vi "initialise.vi"(8 "error in (no error)":errorcluster, 11 "GenericPlugin in":refnum<class "TrajectoryMG100122GenericFPGA.lvclass">) -> (0 "error out":errorcluster, 3 "GenericPlugin out":refnum<class "TrajectoryMG100122GenericFPGA.lvclass">)   [LabVIEW 2010, in "TrajectoryMG100122GenericFPGA.lvclass"]
doc: "The dynamic dispatch-version of this VI initalises the plug-in object by allocating and initalising any dynamic resources need."
uses:
  TrajectoryMG100122GenericFPGA.lvclass
  GenericTrajectory/GenericTrajectory/GenericTrajectory.lvclass
  FPGAWrapper/GenericFPGAWrapper/GenericFPGAWrapper/GenericFPGAWrapper.lvclass
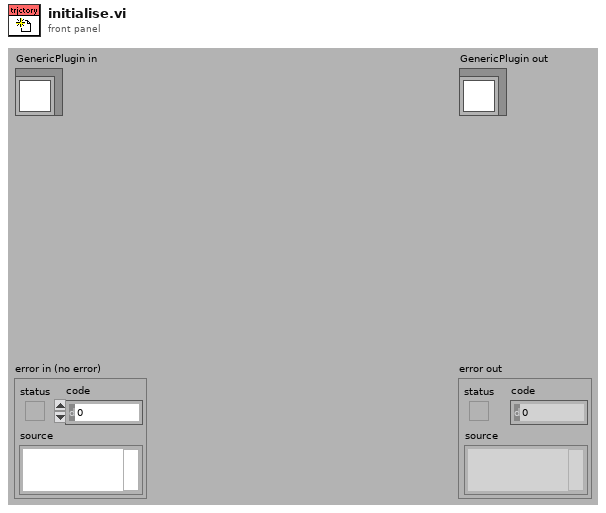
[diagram p1: front panel]
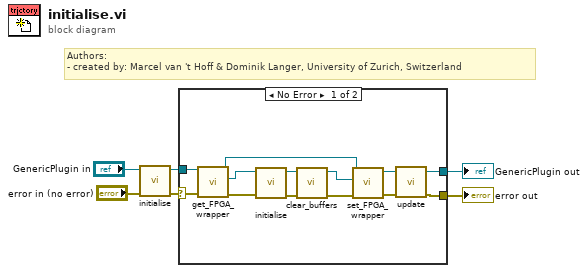
[diagram p0: block diagram]
diagram:
  # "Authors: \n- created by: Marcel van 't Hoff & Dominik Langer, University of Zurich, Switzerland"
  n1 = call-parent "initialise.vi"("error in (no error)"="error in (no error)", "GenericPlugin in"="GenericPlugin in") -> ("error out"=w4:errorcluster, "GenericPlugin out"=w3:refnum<class "TrajectoryMG100122GenericFPGA.lvclass">)  [unwired: 8 in]
  n2 = case shown="No Error" w4 {
    selector: w4 -> [w19 w20]
    tunnel: w3 -> [w18 w21]
    tunnel: [w8 w20] -> w2
    tunnel: [w9 w21] -> w1
    frame No Error {
      n3 = call-dynamic "get_FPGA_wrapper.vi"("error in (no error)"=w19, "TrajectoryMG100122GenericFPGA in"=w18) -> ("error out"=w17:errorcluster, "GenericFPGAWrapper.lvclass"=w16:refnum<class "GenericFPGAWrapper.lvclass">, "TrajectoryMG100122GenericFPGA out"=w15:refnum<class "TrajectoryMG100122GenericFPGA.lvclass">)  [unwired: 7 in]
      n4 = call-dynamic "initialise.vi"("error in (no error)"=w17, "GenericPlugin in"=w16) -> ("error out"=w11:errorcluster, "GenericPlugin out"=w14:refnum<class "GenericFPGAWrapper.lvclass">)  [unwired: 8 in]
      n5 = call-dynamic "clear_buffers.vi"("error in (no error)"=w11, "GenericFPGAWrapper in"=w14) -> ("error out"=w13:errorcluster, "GenericFPGAWrapper out"=w12:refnum<class "GenericFPGAWrapper.lvclass">)  [unwired: 8 in]
      n6 = call-dynamic "set_FPGA_wrapper.vi"("error in (no error)"=w13, "GenericFPGAWrapper.lvclass"=w12, "TrajectoryMG100122GenericFPGA in"=w15) -> ("error out"=w7:errorcluster, "TrajectoryMG100122GenericFPGA out"=w10:refnum<class "TrajectoryMG100122GenericFPGA.lvclass">)  [unwired: 7 in]
      n7 = call-dynamic "update.vi"("error in (no error)"=w7, "TrajectoryMG100122GenericFPGA in"=w10) -> ("error out"=w8:errorcluster, "TrajectoryMG100122GenericFPGA out"=w9:refnum<class "TrajectoryMG100122GenericFPGA.lvclass">)  [unwired: 8 in]
    }
    frame Error {
    }
  }
  "error out" <- w2
  "GenericPlugin out" <- w1
